vi "Base 64 Encode.vi"(5 "Input String":string) -> (1 "?":bool=TRUE, 2 "Output String":string)   [LabVIEW 2011]
panel:
  # "Empty"
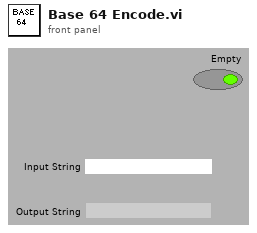
[diagram p1: front panel]
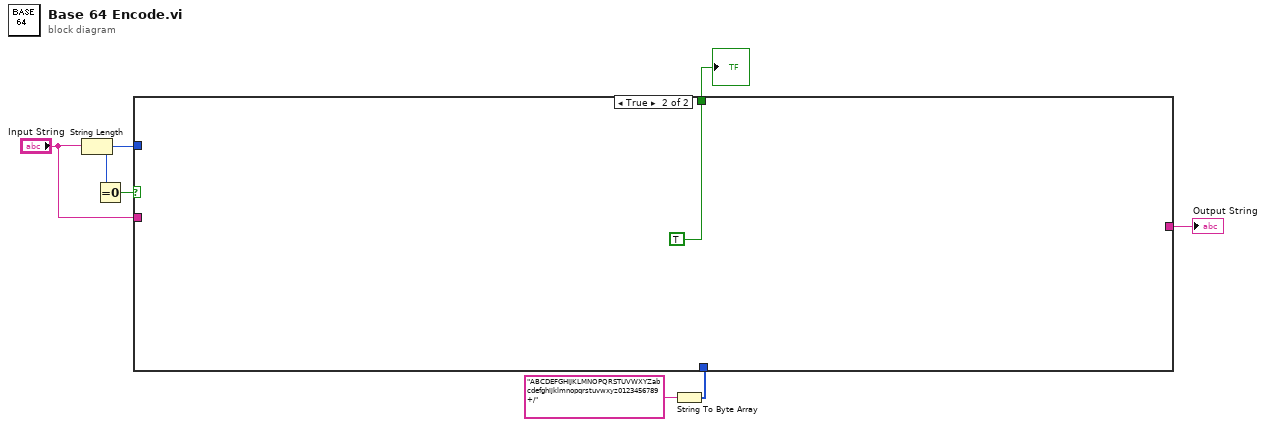
[diagram p0: block diagram]
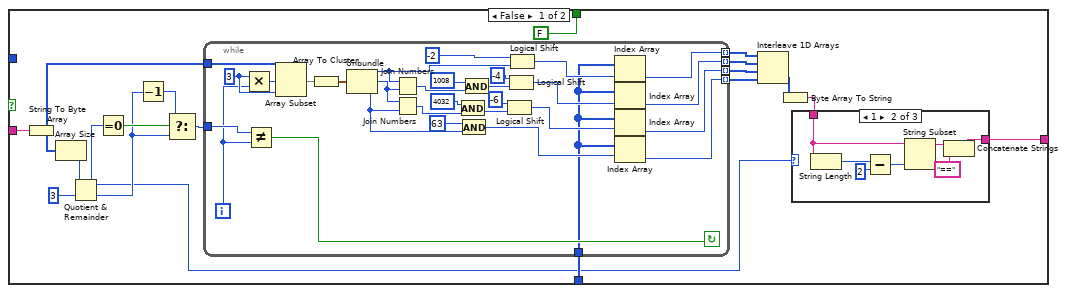
[diagram p2: hidden frame]
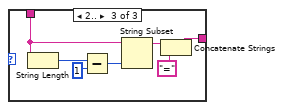
[diagram p4: hidden frame]
diagram:
  n1 = String Length(string="Input String") -> (length=w2:i32)
  n2 = Equal To 0?(x=w2) -> (x = 0?=w3:bool)
  n3 = String To Byte Array(string="ABCDEFGHIJKLMNOPQRSTUVWXYZabcdefghijklmnopqrstuvwxyz0123456789+/") -> (unsigned byte array=w4:u8[])
  n4 = case shown="True" w3 {
    tunnel: [w9 ""] -> w6
    tunnel: "Input String" -> [w18 _]
    tunnel: w2 -> [_ _]
    tunnel: w4 -> [w20 _]
    tunnel: [FALSE TRUE] -> w1
    frame False {
      n5 = String To Byte Array(string=w18) -> (unsigned byte array=w17:u8[])
      n6 = Array Size(array=w17) -> (size(s)=w21:i32)
      n7 = Quotient & Remainder(x=w21, y=3) -> (x-y*floor(x/y)=w10:i32, floor(x/y)=w24:i32)
      n8 = Equal To 0?(x=w10) -> (x = 0?=w25:bool)
      n9 = Decrement(x=w24) -> (x-1=w23:i32)
      n10 = Select(t=w23, s=w25, f=w24) -> (s? t:f=w19:i32)
      n11 = while {
        tunnel: [w26] -> w13 mode=indexing
        tunnel: [w27] -> w14 mode=indexing
        tunnel: [w28] -> w15 mode=indexing
        tunnel: [w29] -> w16 mode=indexing
        tunnel: w19 -> [w50]
        tunnel: w20 -> [w30]
        tunnel: w17 -> [w55]
        i -> [w49]
        stop <- w48 continue-if-true
        w53 = 3 ("x")
        n12 = Multiply(x=w53, y=w49) -> (x*y=w54:i32)
        n13 = Not Equal?(x=w50, y=w49) -> (x != y?=w48:bool)
        n14 = Array Subset(array=w55, index=w54, length=w53) -> (w51:u8[])
        n15 = Array To Cluster(array=w51) -> (cluster=w52:cluster{"[0]":u8, "[1]":u8, "[2]":u8})
        n16 = Unbundle(w52) -> ("[0]"=w37:u8, "[1]"=w42:u8, "[2]"=w36:u8)
        n17 = Join Numbers(hi=w37, lo=w42) -> ((hi.lo)=w46:u16)
        n18 = Join Numbers(hi=w42, lo=w36) -> ((hi.lo)=w41:u16)
        n19 = And(x=u16 4032, y=w41) -> (x .and. y?=w39:u16)
        n20 = And(x=u8 63, y=w36) -> (x .and. y?=w31:u8)
        n21 = And(x=u16 1008, y=w46) -> (x .and. y?=w44:u16)
        n22 = Logical Shift(y=i8 -6, x=w39) -> (x << y=w32:u16)
        n23 = Logical Shift(y=i8 -4, x=w44) -> (x << y=w33:u16)
        n24 = Logical Shift(y=i8 -2, x=w37) -> (x << y=w34:u8)
        n25 = Index Array(array=w30, index=w34) -> (element=w29:u8)
        n26 = Index Array(array=w30, index=w33) -> (element=w28:u8)
        n27 = Index Array(array=w30, index=w32) -> (element=w27:u8)
        n28 = Index Array(array=w30, index=w31) -> (element=w26:u8)
      }
      n29 = Interleave 1D Arrays(w16, w15, w14, w13) -> (w12:u8[])
      n30 = Byte Array To String(unsigned byte array=w12) -> (string=w11:string)
      n31 = case shown="1" w10 {
        tunnel: w11 -> [w56 w58 w65]
        tunnel: [w56 w57 w64] -> w9
        frame ..0 {
        }
        frame 1 {
          n32 = String Length(string=w58) -> (length=w62:i32)
          n33 = Subtract(x=w62, y=i16 2) -> (x-y=w61:i32)
          n34 = String Subset(string=w58, length (rest)=w61) -> (substring=w59:string)  [unwired: 1 in]
          n35 = Concatenate Strings(w59, "==") -> (w57:string)
        }
        frame 2.. {
          n36 = String Length(string=w65) -> (length=w69:i32)
          n37 = Subtract(x=w69, y=i16 1) -> (x-y=w68:i32)
          n38 = String Subset(string=w65, length (rest)=w68) -> (substring=w66:string)  [unwired: 1 in]
          n39 = Concatenate Strings(w66, "=") -> (w64:string)
        }
      }
    }
    frame True {
    }
  }
  "Output String" <- w6
  "?" <- w1
